vi "Mono Helper.vi"(8 "error in (no error)":errorcluster, 9 "no of iterations before stop":i32=20, 10 "wavelength in":dbl, 11 "Monochromator in":refnum<class "Monochromator.lvclass">) -> (0 "error out":errorcluster, 2 "wavelength out":dbl, 3 "Monochromator out":refnum<class "Monochromator.lvclass">)   [LabVIEW 2020, in "Examples.lvlib"]
doc: "Helper VI to move the mono for the CCD examples."
uses:
  Examples.lvlib
  Classes/Mono/Monochromator.lvclass
  8b6ae4ef-647e-49af-919c-4c3e18ac60a9.vi
  0a295a74-6368-4cdc-bef5-bab65824a4b3.vi
panel:
  # "Connector Pane"
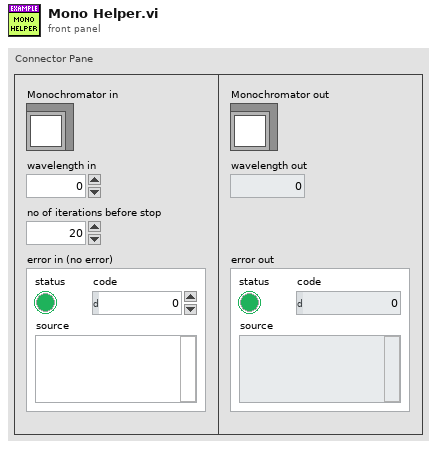
[diagram p1: front panel]
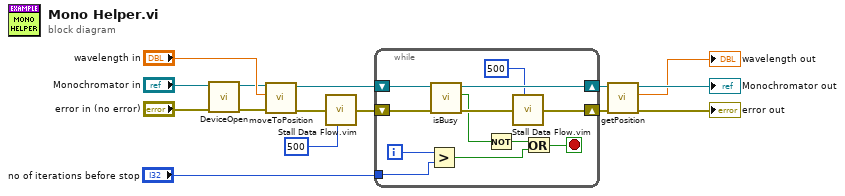
[diagram p0: block diagram]
diagram:
  n1 = call-dynamic "DeviceOpen.vi"("error in (no error)"="error in (no error)", "Monochromator in"="Monochromator in") -> ("error out"=w12:errorcluster, "Monochromator out"=w11:refnum<class "Monochromator.lvclass">)  [unwired: 6 in, 2 out]
  n2 = call "moveToPosition.vi"("error in (no error)"=w12, "wavelength"="wavelength in", "Monochromator in"=w11) -> ("error out"=w4:errorcluster, "Monochromator out"=w7:refnum<class "Monochromator.lvclass">)  [unwired: 5 in, 2 out]
  n3 = call "Stall Data Flow.vim"("value in"=w4, "milliseconds to wait"=u32 500) -> ("value out"=w5:errorcluster)  [unwired: 1 out]
  n4 = while {
    shift-right: [w23] -> w10
    shift-left: w5 -> [w25]
    shift-right: [w26] -> w9
    shift-left: w7 -> [w24]
    tunnel: "no of iterations before stop" -> [w16]
    i -> [w18]
    stop <- w20 stop-if-true
    n5 = Greater?(x=w18, y=w16) -> (0:w17:bool)
    n6 = call "isBusy.vi"("error in (no error)"=w25, "Monochromator in"=w24) -> ("error out"=w27:errorcluster, "mono is busy?"=w21:bool, "Monochromator out"=w26:refnum<class "Monochromator.lvclass">)  [unwired: 7 in]
    n7 = Not(x=w21) -> (.not. x?=w19:bool)
    n8 = call "Stall Data Flow.vim"("value in"=w27, "milliseconds to wait"=u32 500) -> ("value out"=w23:errorcluster)  [unwired: 1 out]
    n9 = Or(x=w19, y=w17) -> (x .or. y?=w20:bool)
  }
  n10 = call "getPosition.vi"("error in (no error)"=w10, "Monochromator in"=w9) -> ("error out"=→"error out":errorcluster, "wavelength"=→"wavelength out":dbl, "Monochromator out"=→"Monochromator out":refnum<class "Monochromator.lvclass">)  [unwired: 7 in]
